vi "StartMeasurement.vi"(0 "Multiharp in":refnum<class "Multiharp.lvclass">, 1 "Coincidence Delays":dbl[](array[numeric]), 2 "Path":path, 5 "tacq":i32, 7 "Max Triggers":i32, 9 "Scanning":bool, 11 "error in (no error)":errorcluster, 12 "Coincidence Window":dbl) -> (4 "Multiharp out":refnum<class "Multiharp.lvclass">, 15 "error out":errorcluster)   [LabVIEW 2023, in "Multiharp.lvlib" / "Multiharp.lvclass"]
uses:
  Multiharp.lvclass
panel:
  in  "event data":T1
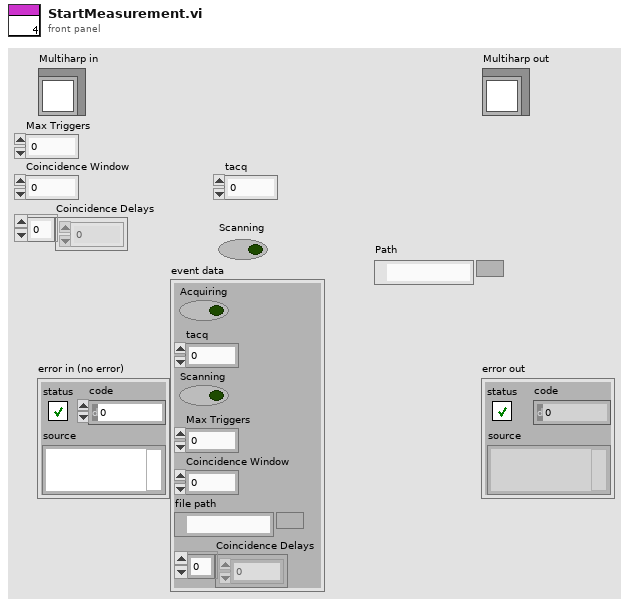
[diagram p1: front panel]
types:
  T1 = cluster{"Acquiring":bool, "tacq":i32, "Scanning":bool, "Max Triggers":i32, "Coincidence Window":dbl, "file path":path, "Coincidence Delays":dbl[]}
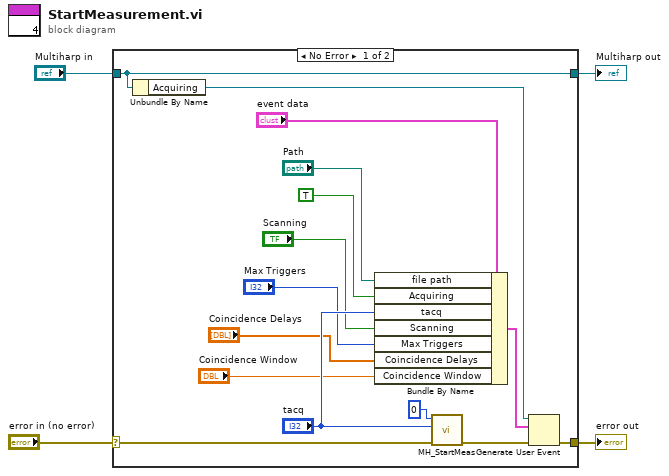
[diagram p0: block diagram]
diagram:
  n1 = case shown="No Error" "error in (no error)" {
    selector: "error in (no error)" -> [w11 w21]
    tunnel: [w17 w21] -> w3
    tunnel: [w19 w20] -> w1
    tunnel: "Multiharp in" -> [w19 w20]
    frame No Error {
      n2 = Unbundle By Name(w19) -> ("Acquiring"=w18:refnum<user-event>)
      n3 = Bundle By Name(cluster="event data", "file path"="Path", "Acquiring"=TRUE, "tacq"="tacq", "Scanning"="Scanning", "Max Triggers"="Max Triggers", "Coincidence Delays"="Coincidence Delays", "Coincidence Window"="Coincidence Window") -> (w6:T1)
      n4 = call "MH_StartMeas.vi"("error in (no error)"=w11, "tacq"="tacq", "devidx"=0) -> ("error out"=w14:errorcluster)  [unwired: 7 in, 1 out]
      n5 = Generate User Event(user event=w18, event data cluster=w6, error in=w14) -> (error out=w17:errorcluster)  [unwired: 1 in, 1 out]
    }
    frame Error {
    }
  }
  "error out" <- w3
  "Multiharp out" <- w1
